vi "Init Events.vi"(8 "error in (no error)":errorcluster, 11 "Temp01 in":refnum<class "TELLC_Temp01.lvclass">) -> (0 "error out":errorcluster, 3 "Temp01 out":refnum<class "TELLC_Temp01.lvclass">)   [LabVIEW 2017, in "TELLC_Temp01.lvclass"]
doc: "Developed by Kevin Thompson\nkevin@thompsonengineering.net\n\nCopyright 2018\nThompson Engineering, LLC"
uses:
  TELLC_Temp01.lvclass
  Common/DataTypes/TD Async CmdMsg EventData--cluster.ctl
  TELLC_Temp01.lvclass/TELLC_Temp01.ctl
  Accessors/Get PublicEvents.vi
  Accessors/Set PublicEvents.vi
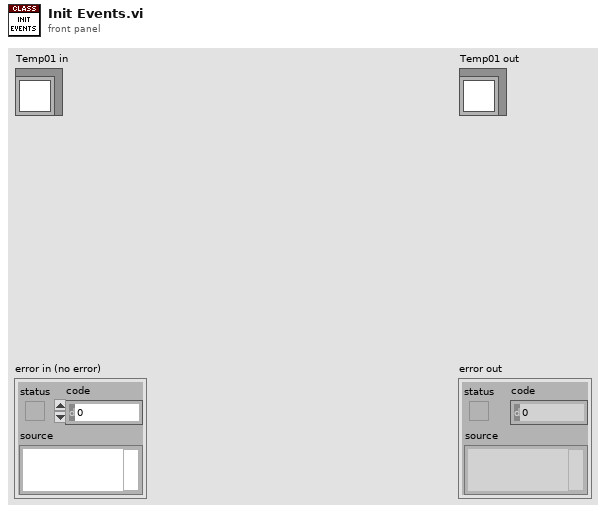
[diagram p1: front panel]
types:
  T1 = typedef "TD Async CmdMsg EventData--cluster.ctl" = cluster{"Time Stamp":timestamp, "CmdMsg":string, "vData":variant}
  T2 = typedef "TELLC_Temp01.lvclass/Public Events--cluster.ctl" = cluster{"Temp01.AsyncCmd Event":refnum<user-event>, "Temp01.AsyncMsg Event":refnum<user-event>, "stop process":refnum<user-event>}
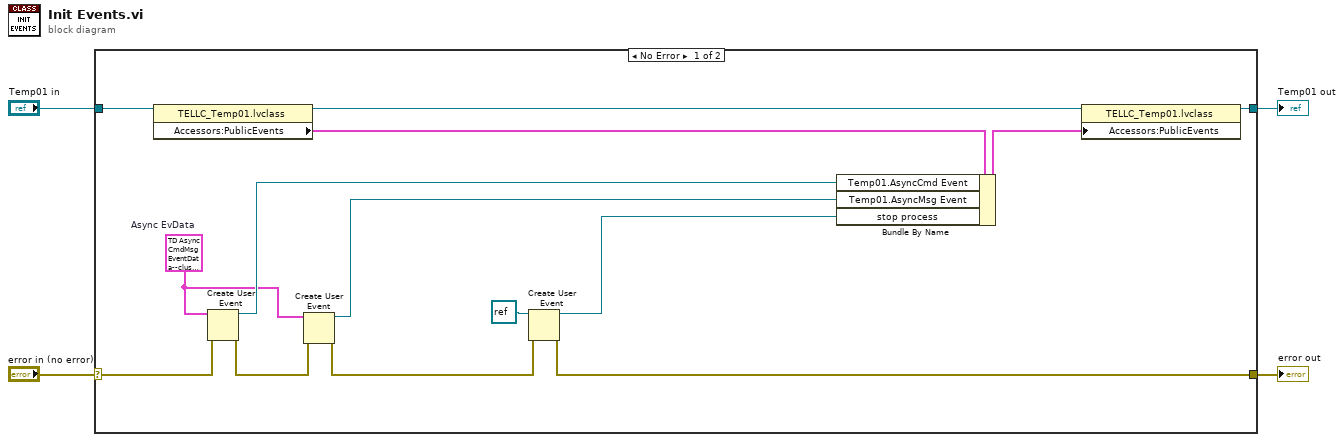
[diagram p0: block diagram]
diagram:
  n1 = case shown="No Error" "error in (no error)" {
    selector: "error in (no error)" -> [w9 w20]
    tunnel: [w10 w20] -> w3
    tunnel: [w18 w19] -> w1
    tunnel: "Temp01 in" -> [w17 w19]
    frame No Error {
      w6 = T1 {"Time Stamp"=timestamp(0 s since 1904-01-01), "CmdMsg"="", "vData"=variant}  # Async EvData
      n2 = property class="TELLC_Temp01.lvclass"(reference=w17) -> (reference out=w16:refnum<class "TELLC_Temp01.lvclass">, "Accessors:PublicEvents"=w15:T2)  [unwired: 1 in, 1 out]
      n3 = Create User Event(user event datatype=w6, error in=w9) -> (user event=w11:refnum<user-event>, error out=w8:errorcluster)
      n4 = Create User Event(user event datatype=w6, error in=w8) -> (user event=w5:refnum<user-event>, error out=w7:errorcluster)
      n5 = Create User Event(user event datatype=refnum<notifier> refnum ("notifier out"), error in=w7) -> (user event=w12:refnum<user-event>, error out=w10:errorcluster)
      n6 = Bundle By Name(cluster=w15, "Temp01.AsyncCmd Event"=w11, "Temp01.AsyncMsg Event"=w5, "stop process"=w12) -> (w14:T2)
      n7 = property class="TELLC_Temp01.lvclass"(reference=w16, "Accessors:PublicEvents"=w14) -> (reference out=w18:refnum<class "TELLC_Temp01.lvclass">)  [unwired: 1 in, 1 out]
    }
    frame Error {
    }
  }
  "error out" <- w3
  "Temp01 out" <- w1
